vi "U8 to BCD.vi"(11 "decimal in":u8) -> (2 "low nibble":u8, 3 "hi nibble":u8)   [LabVIEW 2020]
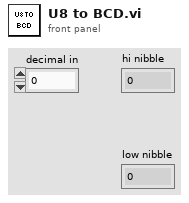
[diagram p1: front panel]
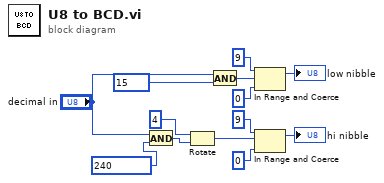
[diagram p0: block diagram]
diagram:
  n1 = And(x="decimal in", y=u8 240) -> (x .and. y?=w6:u8)
  n2 = Rotate(1:w6, 2:i16 4 ("y")) -> (0:w12:u8)
  n3 = And(x="decimal in", y=u8 15) -> (x .and. y?=w13:u8)
  n4 = In Range and Coerce(upper limit=u8 9, x=w13, lower limit=u8 0) -> (coerced(x)=→"low nibble":u8)  [unwired: 1 out]
  n5 = In Range and Coerce(upper limit=u8 9, x=w12, lower limit=u8 0) -> (coerced(x)=→"hi nibble":u8)  [unwired: 1 out]
